vi "Shut Down Device.vi"(8 "error in (no error)":errorcluster, 11 "Arduino DAQ in":refnum<class "Arduino DAQ.lvclass">) -> (0 "error out":errorcluster, 3 "Arduino DAQ out":refnum<class "Arduino DAQ.lvclass">)   [LabVIEW 2023, in "Arduino DAQ.lvlib" / "Arduino DAQ.lvclass"]
uses:
  Arduino DAQ.lvclass
  Arduino DAQ.lvclass/Arduino DAQ.ctl
  Sync Device/Sync Device.lvclass
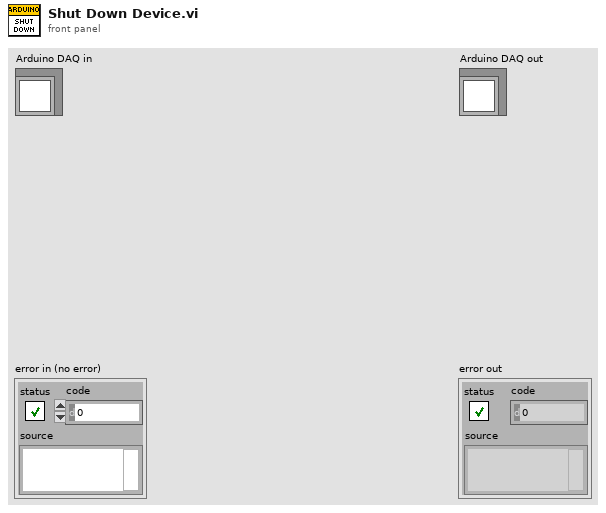
[diagram p1: front panel]
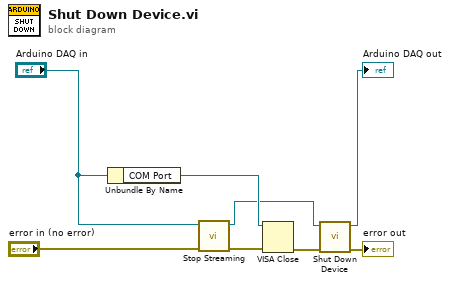
[diagram p0: block diagram]
diagram:
  n1 = Unbundle By Name("Arduino DAQ in") -> ("COM Port"=w3:refnum<visa-resource-name>)
  n2 = call-dynamic "Stop Streaming.vi"("error in (no error)"="error in (no error)", "Synchronization Device in"="Arduino DAQ in") -> ("error out"=w4:errorcluster, "Synchronization Device out"=w1:refnum<class "Arduino DAQ.lvclass">)  [unwired: 8 in]
  n3 = VISA Close(VISA resource name=w3, error in (no error)=w4) -> (error out=w6:errorcluster)
  n4 = call-parent "Shut Down Device.vi"("error in (no error)"=w6, "Device in"=w1) -> ("error out"=→"error out":errorcluster, "Device out"=→"Arduino DAQ out":refnum<class "Arduino DAQ.lvclass">)  [unwired: 8 in]
